vi "M-227 Control.vi"(0 "M-227 Notifier":refnum<notifier>, 5 "Stage Action":T1={"Action"=enum."Get Position", "Axis"=[], "Setpoint"=[], "Velocity"=0.5, "Cmd Recvd?"=FALSE, "Position"=[], "Status"=enum."Error", "Misc"=variant} {"Velocity" min=0.0 max=1.0 step=0.01}, 11 "VISA In":refnum<visa-resource-name>) -> (4 "M-227 Notifier (Dup)":refnum<notifier>)   [LabVIEW 2016]
uses:
  Stages Controls/Stage Notifier Element.ctl
  Stages Controls/Stage Actions.ctl
  Stages Controls/Stage Status.ctl
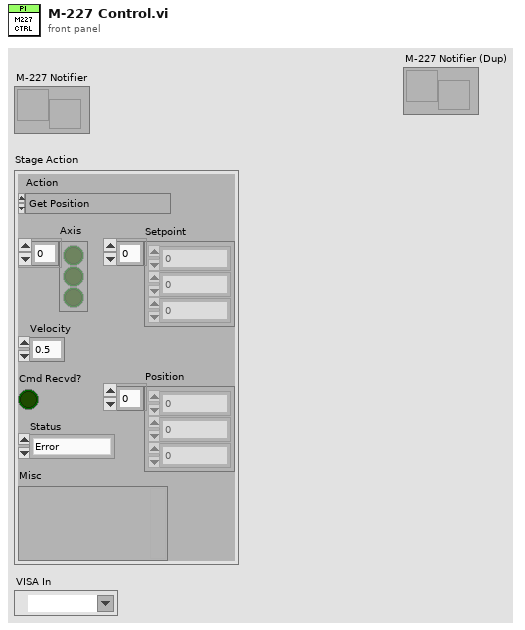
[diagram p1: front panel]
types:
  T1 = typedef "Stage Notifier Element.ctl" = cluster{"Action":T2, "Axis":bool[], "Setpoint":dbl[], "Velocity":dbl, "Cmd Recvd?":bool, "Position":dbl[], "Status":T3, "Misc":variant}
  T2 = typedef "Stage Actions.ctl" = enum16{"Get Position", "MVR", "SVR", "MOVE", "SVA", "HALT", "ONTARGET", "ERROR", "REFERENCE", "INIT", "VELOCITY", "STATUS", "EXIT", "HOME", "ZEROPOS", "NANOPOS", "ANALOG", "QUIT"}
  T3 = typedef "Stage Status.ctl" = enum16{"Error", "Abort", "Busy", "On Target"}
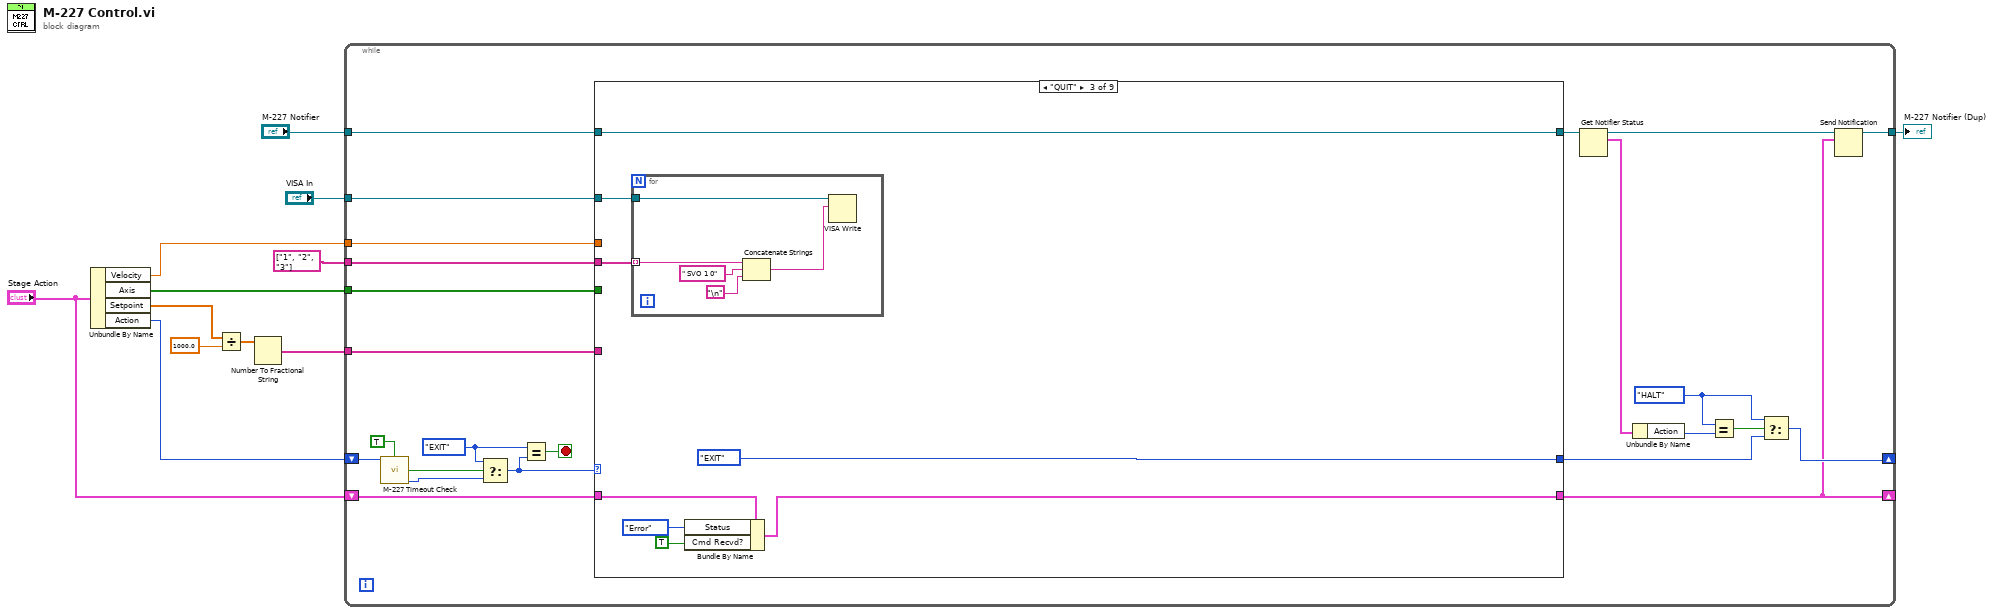
[diagram p0: block diagram]
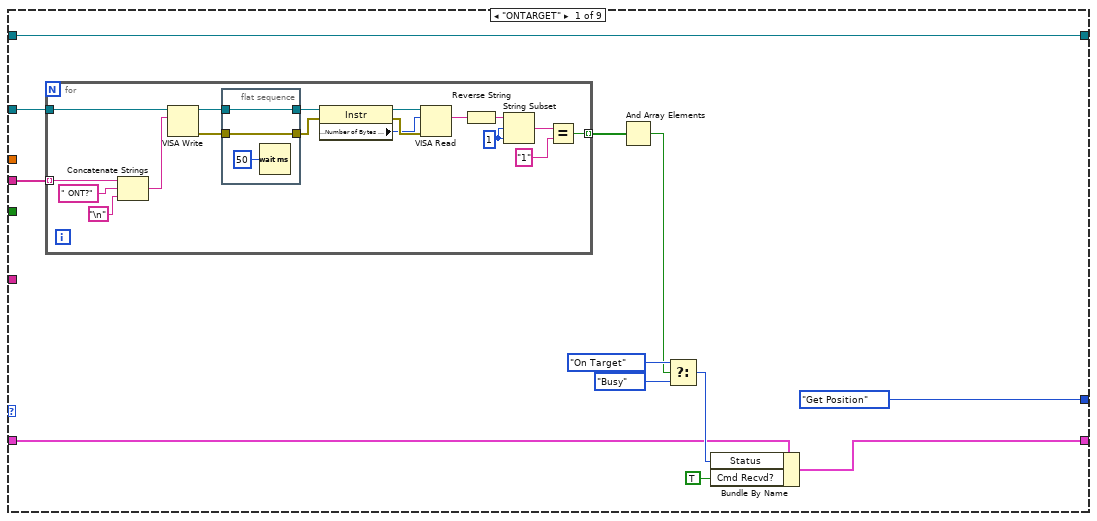
[diagram p2: hidden frame]
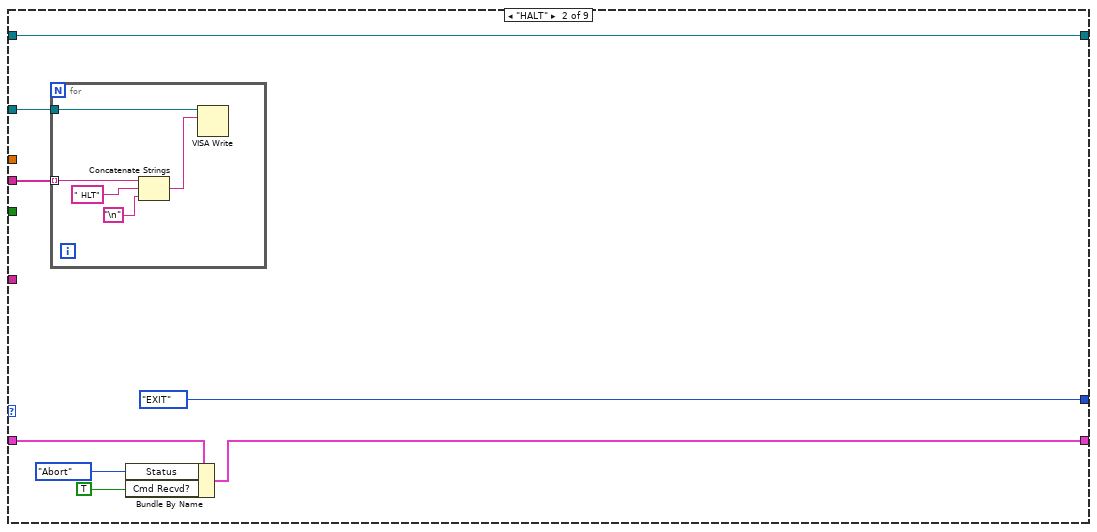
[diagram p3: hidden frame]
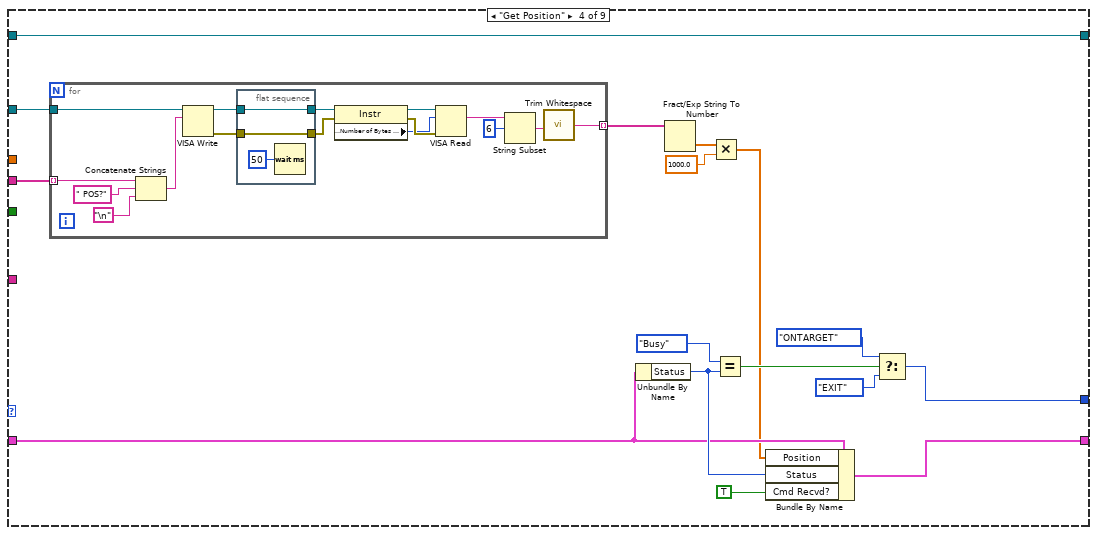
[diagram p4: hidden frame]
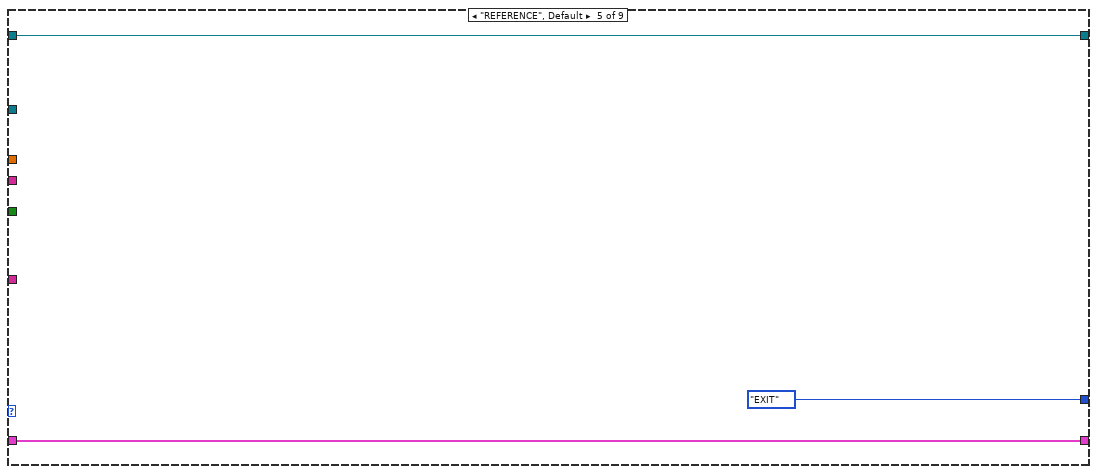
[diagram p5: hidden frame]
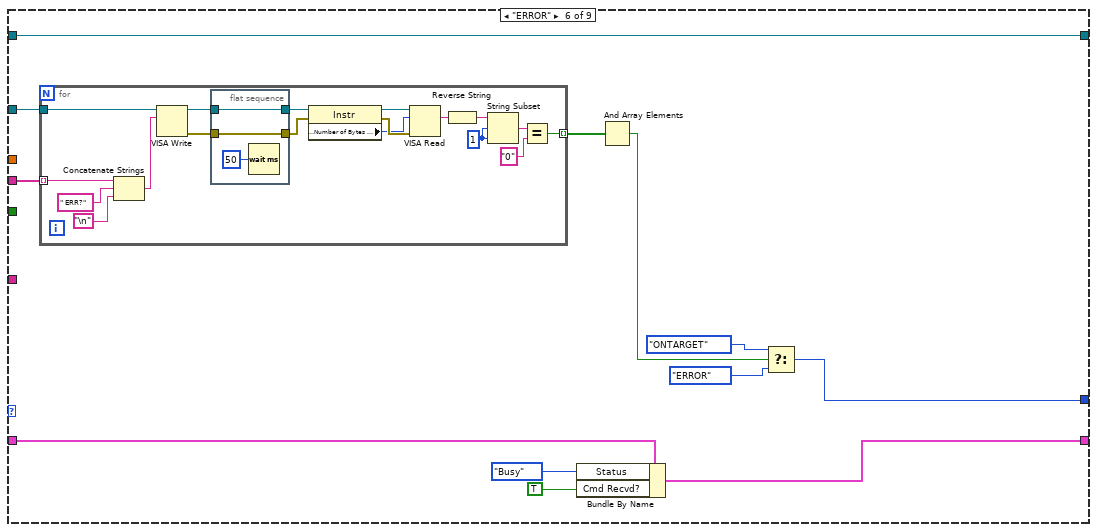
[diagram p6: hidden frame]
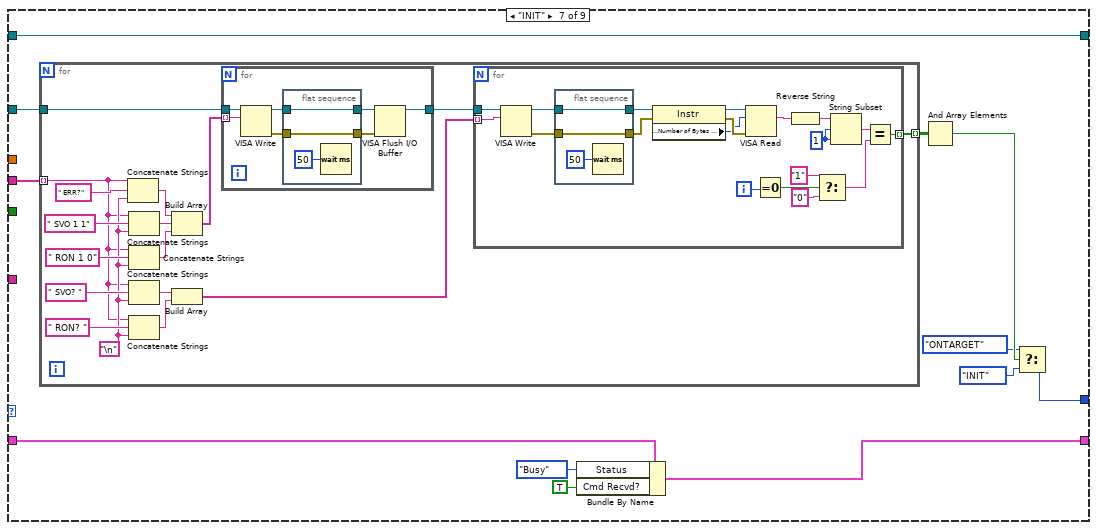
[diagram p7: hidden frame]
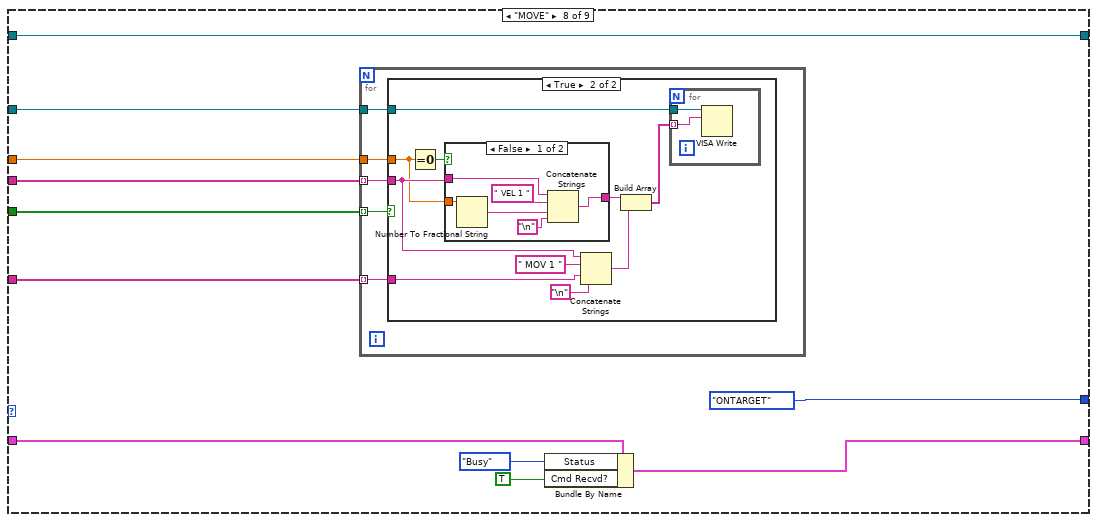
[diagram p8: hidden frame]
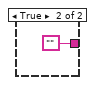
[diagram p10: hidden frame]
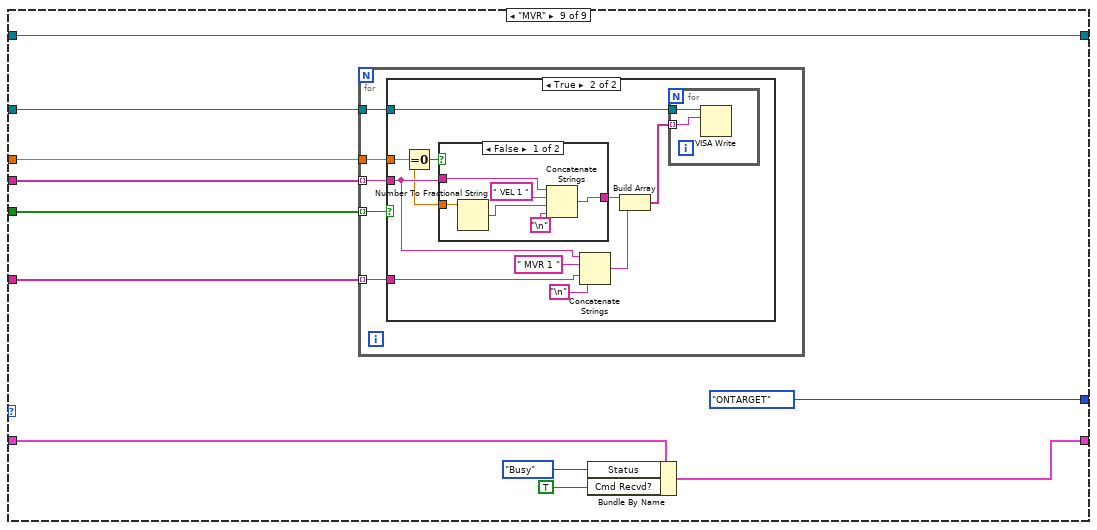
[diagram p11: hidden frame]
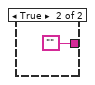
[diagram p13: hidden frame]
diagram:
  n1 = Unbundle By Name("Stage Action") -> ("Velocity"=w9:dbl, "Axis"=w8:bool[], "Setpoint"=w5:dbl[], "Action"=w7:T2)
  n2 = Divide(x=w5, y=1000.0) -> (x/y=w6:dbl[])
  n3 = Number To Fractional String(number=w6) -> (F-format string=w10:string[])  [unwired: 3 in]
  n4 = while {
    tunnel: string[] ["1", "2", "3"] -> [w36]
    tunnel: "VISA In" -> [w35]
    shift-right: [w30] -> _
    shift-left: w7 -> [w27]
    tunnel: w8 -> [w33]
    tunnel: w9 -> [w32]
    tunnel: w10 -> [w34]
    shift-right: [w29] -> _
    shift-left: "Stage Action" -> [w31]
    tunnel: "M-227 Notifier" -> [w15]
    tunnel: [w13] -> w1
    stop <- w23 stop-if-true
    w17 = Stage_Actions."HALT" ("Action")
    w26 = Stage_Actions."EXIT" ("t")
    n5 = call "M-227 Timeout Check.vi"("Action"=w27, "User Input?"=TRUE) -> ("Timeout?"=w24:bool, "Action (Dup)"=w25:T2)  [unwired: 12 in]
    n6 = Select(t=w26, s=w24, f=w25) -> (s? t:f=w21:T2)
    n7 = Equal?(x=w26, y=w21) -> (x = y?=w23:bool)
    n8 = case shown="\"QUIT\"" w21 {
      tunnel: w36 -> [w48 w77 w90 w111 _ w145 w178 w238 w273]
      tunnel: w35 -> [w38 w71 w84 w97 _ w134 w167 w229 w264]
      tunnel: w34 -> [_ _ _ _ _ _ _ w237 w272]
      tunnel: w33 -> [_ _ _ _ _ _ _ w236 w271]
      tunnel: w32 -> [_ _ _ _ _ _ _ w235 w270]
      tunnel: [Stage_Actions."Get Position" ("Action") Stage_Actions."EXIT" ("Action") Stage_Actions."EXIT" ("Action") w103 Stage_Actions."EXIT" ("Action") w137 w170 Stage_Actions."ONTARGET" ("Action") Stage_Actions."ONTARGET" ("Action")] -> w28
      tunnel: w31 -> [w39 w73 w86 w102 w132 w141 w174 w231 w265]
      tunnel: [w42 w72 w85 w101 w132 w142 w175 w230 w266] -> w29
      tunnel: w15 -> [w37 w70 w83 w96 w131 w135 w168 w228 w263]
      tunnel: [w37 w70 w83 w96 w131 w135 w168 w228 w263] -> w14
      frame "ONTARGET" {
        n9 = for {
          tunnel: w48 -> [w66] mode=indexing
          tunnel: [w65] -> w47 mode=indexing
          tunnel: w38 -> [w49]
          w61 = 1 ("length (rest)")
          n10 = Concatenate Strings(w66, " ONT?" ("string"), "\n") -> (w53:string)
          n11 = VISA Write(VISA resource name=w49, write buffer=w53) -> (VISA resource name out=w60:refnum<visa-resource-name>, error out=w59:errorcluster)  [unwired: 1 in, 1 out]
          n12 = flat-sequence {
            tunnel: w60 -> [w68]
            tunnel: w59 -> [w67]
            tunnel: [w68] -> w58
            tunnel: [w67] -> w57
            frame #0 {
              n13 = Wait (ms)(milliseconds to wait=u32 50) -> ()  [unwired: 1 out]
            }
          }
          n14 = property class="Instr"(reference=w58, error in=w57) -> (reference out=w56:refnum<visa-resource-name>, error out=w55:errorcluster, "Serial Settings:Number of Bytes at Serial Port"=w54:u32)
          n15 = VISA Read(VISA resource name=w56, byte count=w54, error in (no error)=w55) -> (read buffer=w52:string)  [unwired: 3 out]
          n16 = Reverse String(1:w52) -> (0:w62:string)
          n17 = String Subset(string=w62, offset (0)=w61, length (rest)=w61) -> (substring=w51:string)
          n18 = Equal?(x=w51, y="1") -> (x = y?=w65:bool)
        }
        n19 = And Array Elements(Boolean array=w47) -> (logical AND=w40:bool)
        n20 = Select(t=Stage_Status."On Target" ("Status"), s=w40, f=Stage_Status."Busy" ("Status")) -> (s? t:f=w41:T3)
        n21 = Bundle By Name(cluster=w39, "Status"=w41, "Cmd Recvd?"=TRUE) -> (w42:T1)
      }
      frame "HALT" {
        n22 = for {
          tunnel: w77 -> [w81] mode=indexing
          tunnel: w71 -> [w78]
          n23 = Concatenate Strings(w81, " HLT" ("string"), "\n") -> (w80:string)
          n24 = VISA Write(VISA resource name=w78, write buffer=w80) -> ()  [unwired: 1 in, 3 out]
        }
        n25 = Bundle By Name(cluster=w73, "Status"=Stage_Status."Abort", "Cmd Recvd?"=TRUE) -> (w72:T1)
      }
      frame "QUIT" {
        n26 = for {
          tunnel: w90 -> [w93] mode=indexing
          tunnel: w84 -> [w91]
          n27 = Concatenate Strings(w93, " SVO 1 0" ("string"), "\n") -> (w92:string)
          n28 = VISA Write(VISA resource name=w91, write buffer=w92) -> ()  [unwired: 1 in, 3 out]
        }
        n29 = Bundle By Name(cluster=w86, "Status"=Stage_Status."Error", "Cmd Recvd?"=TRUE) -> (w85:T1)
      }
      frame "Get Position" {
        n30 = for {
          tunnel: w111 -> [w127] mode=indexing
          tunnel: [w126] -> w110 mode=indexing
          tunnel: w97 -> [w112]
          n31 = Concatenate Strings(w127, " POS?" ("string"), "\n") -> (w114:string)
          n32 = VISA Write(VISA resource name=w112, write buffer=w114) -> (VISA resource name out=w121:refnum<visa-resource-name>, error out=w120:errorcluster)  [unwired: 1 in, 1 out]
          n33 = flat-sequence {
            tunnel: w121 -> [w129]
            tunnel: w120 -> [w128]
            tunnel: [w129] -> w119
            tunnel: [w128] -> w118
            frame #0 {
              n34 = Wait (ms)(milliseconds to wait=u32 50) -> ()  [unwired: 1 out]
            }
          }
          n35 = property class="Instr"(reference=w119, error in=w118) -> (reference out=w117:refnum<visa-resource-name>, error out=w116:errorcluster, "Serial Settings:Number of Bytes at Serial Port"=w115:u32)
          n36 = VISA Read(VISA resource name=w117, byte count=w115, error in (no error)=w116) -> (read buffer=w113:string)  [unwired: 3 out]
          n37 = String Subset(string=w113, offset (0)=6) -> (substring=w122:string)  [unwired: 1 in]
          n38 = call <vilib>:"Trim Whitespace.vi"("string"=w122) -> ("trimmed string"=w126:string)  [unwired: 1 in]
        }
        n39 = Unbundle By Name(w102) -> ("Status"=w106:T3)
        n40 = Fract/Exp String To Number(string=w110) -> (number=w100:dbl[])  [unwired: 3 in, 1 out]
        n41 = Multiply(x=w100, y=1000.0) -> (x*y=w99:dbl[])
        n42 = Equal?(x=Stage_Status."Busy", y=w106) -> (x = y?=w107:bool)
        n43 = Bundle By Name(cluster=w102, "Position"=w99, "Status"=w106, "Cmd Recvd?"=TRUE) -> (w101:T1)
        n44 = Select(t=Stage_Actions."ONTARGET" ("Action"), s=w107, f=Stage_Actions."EXIT" ("Action")) -> (s? t:f=w103:T2)
      }
      frame "REFERENCE", Default {
      }
      frame "ERROR" {
        n45 = for {
          tunnel: w145 -> [w154] mode=indexing
          tunnel: [w147] -> w140 mode=indexing
          tunnel: w134 -> [w146]
          w151 = 1 ("length (rest)")
          n46 = Concatenate Strings(w154, " ERR?" ("string"), "\n") -> (w153:string)
          n47 = VISA Write(VISA resource name=w146, write buffer=w153) -> (VISA resource name out=w163:refnum<visa-resource-name>, error out=w162:errorcluster)  [unwired: 1 in, 1 out]
          n48 = flat-sequence {
            tunnel: w163 -> [w165]
            tunnel: w162 -> [w164]
            tunnel: [w165] -> w161
            tunnel: [w164] -> w160
            frame #0 {
              n49 = Wait (ms)(milliseconds to wait=u32 50) -> ()  [unwired: 1 out]
            }
          }
          n50 = property class="Instr"(reference=w161, error in=w160) -> (reference out=w159:refnum<visa-resource-name>, error out=w158:errorcluster, "Serial Settings:Number of Bytes at Serial Port"=w157:u32)
          n51 = VISA Read(VISA resource name=w159, byte count=w157, error in (no error)=w158) -> (read buffer=w150:string)  [unwired: 3 out]
          n52 = Reverse String(1:w150) -> (0:w152:string)
          n53 = String Subset(string=w152, offset (0)=w151, length (rest)=w151) -> (substring=w149:string)
          n54 = Equal?(x=w149, y="0") -> (x = y?=w147:bool)
        }
        n55 = Bundle By Name(cluster=w141, "Status"=Stage_Status."Busy", "Cmd Recvd?"=TRUE) -> (w142:T1)
        n56 = And Array Elements(Boolean array=w140) -> (logical AND=w139:bool)
        n57 = Select(t=Stage_Actions."ONTARGET" ("Action"), s=w139, f=Stage_Actions."ERROR" ("Action")) -> (s? t:f=w137:T2)
      }
      frame "INIT" {
        n58 = for {
          tunnel: w178 -> [w181] mode=indexing
          tunnel: [w185] -> w173 mode=indexing
          tunnel: w167 -> [w180]
          w182 = "\n"
          n59 = Concatenate Strings(w181, " ERR?" ("string"), w182) -> (w183:string)
          n60 = Concatenate Strings(w181, " SVO 1 1" ("string"), w182) -> (w194:string)
          n61 = Concatenate Strings(w181, " RON 1 0" ("string"), w182) -> (w195:string)
          n62 = Concatenate Strings(w181, " SVO? " ("string"), w182) -> (w192:string)
          n63 = Concatenate Strings(w181, " RON? " ("string"), w182) -> (w193:string)
          n64 = Build Array(w183, w194, w195) -> (w186:string[])
          n65 = Build Array(w192, w193) -> (w187:string[])
          n66 = for {
            tunnel: w186 -> [w202] mode=indexing
            tunnel: w180 -> [w197]
            tunnel: [w196] -> w179
            n67 = VISA Write(VISA resource name=w197, write buffer=w202) -> (VISA resource name out=w200:refnum<visa-resource-name>, error out=w199:errorcluster)  [unwired: 1 in, 1 out]
            n68 = flat-sequence {
              tunnel: w200 -> [w204]
              tunnel: w199 -> [w203]
              tunnel: [w204] -> w201
              tunnel: [w203] -> w198
              frame #0 {
                n69 = Wait (ms)(milliseconds to wait=u32 50) -> ()  [unwired: 1 out]
              }
            }
            n70 = VISA Flush I/O Buffer(VISA resource name=w201, error in (no error)=w198) -> (VISA resource name out=w196:refnum<visa-resource-name>)  [unwired: 1 in, 1 out]
          }
          n71 = for {
            tunnel: w187 -> [w217] mode=indexing
            tunnel: [w212] -> w185 mode=indexing
            tunnel: w179 -> [w206]
            i -> [w208]
            w215 = 1 ("length (rest)")
            n72 = VISA Write(VISA resource name=w206, write buffer=w217) -> (VISA resource name out=w224:refnum<visa-resource-name>, error out=w223:errorcluster)  [unwired: 1 in, 1 out]
            n73 = flat-sequence {
              tunnel: w224 -> [w226]
              tunnel: w223 -> [w225]
              tunnel: [w226] -> w222
              tunnel: [w225] -> w221
              frame #0 {
                n74 = Wait (ms)(milliseconds to wait=u32 50) -> ()  [unwired: 1 out]
              }
            }
            n75 = property class="Instr"(reference=w222, error in=w221) -> (reference out=w220:refnum<visa-resource-name>, error out=w219:errorcluster, "Serial Settings:Number of Bytes at Serial Port"=w218:u32)
            n76 = VISA Read(VISA resource name=w220, byte count=w218, error in (no error)=w219) -> (read buffer=w213:string)  [unwired: 3 out]
            n77 = Equal To 0?(x=w208) -> (x = 0?=w207:bool)
            n78 = Reverse String(1:w213) -> (0:w214:string)
            n79 = Select(t="1", s=w207, f="0") -> (s? t:f=w210:string)
            n80 = String Subset(string=w214, offset (0)=w215, length (rest)=w215) -> (substring=w216:string)
            n81 = Equal?(x=w216, y=w210) -> (x = y?=w212:bool)
          }
        }
        n82 = Bundle By Name(cluster=w174, "Status"=Stage_Status."Busy", "Cmd Recvd?"=TRUE) -> (w175:T1)
        n83 = And Array Elements(Boolean array=w173) -> (logical AND=w172:bool)
        n84 = Select(t=Stage_Actions."ONTARGET" ("Action"), s=w172, f=Stage_Actions."INIT" ("Action")) -> (s? t:f=w170:T2)
      }
      frame "MOVE" {
        n85 = for {
          tunnel: w238 -> [w243] mode=indexing
          tunnel: w237 -> [w242] mode=indexing
          tunnel: w236 -> [w241] mode=indexing
          tunnel: w235 -> [w240]
          tunnel: w229 -> [w239]
          n86 = case shown="True" w241 {
            tunnel: w243 -> [_ w251]
            tunnel: w242 -> [_ w250]
            tunnel: w239 -> [_ w244]
            tunnel: w240 -> [_ w245]
            frame False {
            }
            frame True {
              n87 = Equal To 0?(x=w245) -> (x = 0?=w249:bool)
              n88 = case shown="False" w249 {
                tunnel: w251 -> [w259 _]
                tunnel: [w258 ""] -> w248
                tunnel: w245 -> [w256 _]
                frame False {
                  n89 = Number To Fractional String(number=w256) -> (F-format string=w257:string)  [unwired: 3 in]
                  n90 = Concatenate Strings(w259, " VEL 1 ", w257, "\n") -> (w258:string)
                }
                frame True {
                }
              }
              n91 = Concatenate Strings(w251, " MOV 1 ", w250, "\n") -> (w247:string)
              n92 = Build Array(w248, w247) -> (w246:string[])
              n93 = for {
                tunnel: w246 -> [w255] mode=indexing
                tunnel: w244 -> [w254]
                n94 = VISA Write(VISA resource name=w254, write buffer=w255) -> ()  [unwired: 1 in, 3 out]
              }
            }
          }
        }
        n95 = Bundle By Name(cluster=w231, "Status"=Stage_Status."Busy", "Cmd Recvd?"=TRUE) -> (w230:T1)
      }
      frame "MVR" {
        n96 = for {
          tunnel: w273 -> [w278] mode=indexing
          tunnel: w272 -> [w277] mode=indexing
          tunnel: w271 -> [w276] mode=indexing
          tunnel: w270 -> [w275]
          tunnel: w264 -> [w274]
          n97 = case shown="True" w276 {
            tunnel: w278 -> [_ w286]
            tunnel: w277 -> [_ w285]
            tunnel: w275 -> [_ w284]
            tunnel: w274 -> [_ w279]
            frame False {
            }
            frame True {
              n98 = Equal To 0?(x=w284) -> (x = 0?=w283:bool)
              n99 = case shown="False" w283 {
                tunnel: w286 -> [w294 _]
                tunnel: w284 -> [w292 _]
                tunnel: [w293 ""] -> w282
                frame False {
                  n100 = Number To Fractional String(number=w292) -> (F-format string=w291:string)  [unwired: 3 in]
                  n101 = Concatenate Strings(w294, " VEL 1 ", w291, "\n") -> (w293:string)
                }
                frame True {
                }
              }
              n102 = Concatenate Strings(w286, " MVR 1 ", w285, "\n") -> (w281:string)
              n103 = Build Array(w282, w281) -> (w280:string[])
              n104 = for {
                tunnel: w280 -> [w290] mode=indexing
                tunnel: w279 -> [w289]
                n105 = VISA Write(VISA resource name=w289, write buffer=w290) -> ()  [unwired: 1 in, 3 out]
              }
            }
          }
        }
        n106 = Bundle By Name(cluster=w265, "Status"=Stage_Status."Busy", "Cmd Recvd?"=TRUE) -> (w266:T1)
      }
    }
    n107 = Get Notifier Status(notifier=w14) -> (notifier out=w20:refnum<notifier>, current notification=w16:T1)  [unwired: 1 in, 3 out]
    n108 = Unbundle By Name(w16) -> ("Action"=w18:T2)
    n109 = Equal?(x=w17, y=w18) -> (x = y?=w19:bool)
    n110 = Select(t=w17, s=w19, f=w28) -> (s? t:f=w30:T2)
    n111 = Send Notification(notification=w29, notifier=w20) -> (notifier out=w13:refnum<notifier>)  [unwired: 1 in, 1 out]
  }
  "M-227 Notifier (Dup)" <- w1
